vi "ArrayPadraoSuper.vi"(1 "VI":path, 3 "Array_TAGS/Config":string[](array[string])=["KPS-EVC-001", "KPS-EVC-002", "KPS-EVC-003", "KPS-EVC-004", "KPS-EVC-005", "KPS-EVC-006", "KPS-EVC-007", "KPS-EVC-008", "WPS-EVC-001", "WPS-EVC-002", "WPS-EVC-003", "WPS-EVC-004", "WPS-EVC-005", "WPS-EVC-006", "WPS-EVC-007", "WPS-EVC-008", "AMS-EVC-001B", "AMS-EVC-003A", "FIS-EVC-031", "FIS-EVC-011", "FIS-EVC-012", "FIS-EVC-021", "FIS-EVC-022", "FIS-EVC-001", "FIS-EVC-002", "KMS-EVC-001", "WMS-EVC-001A", "WMS-EVC-001B", "AMS-EVC-001C", "DG-EVC-001", "DG-EVC-ALL", "KPS-WR-ON", "WPS-WR-ON", "KPS-WR-OFF", "WPS-WR-OFF", "AMS-EVC-001A", "AMS-PY-005A", "AMS-FY-004A", "WMS-FCV-001", "KMS-FCV-001", "SPK-WR-VEL", "SPW-WR-VEL", "SKM-FIC-COR-KF-MAX", "SKM-FIC-COR-KF-MIN", "SKM-FIC-COR-WF-MAX", "SKM-FIC-COR-WF-MIN", "FSS-EVC-801", "FSS-EVC-802", "FSS-EVC-803", "CP-Y-601D", "CP-Y-601H", "FSS-EVC-804", "SHD-CV-HD", "SHD-CV-ALV", "SHD-ON-OFF", "FSS-EVC-805", "FSS-EVC-806", "DG-FCV-801", "Aplicação apenas de Leitura ??", "SALVAR/AQUISITAR", "KPS-FCV-001-W", "WPS-FCV-001-W"]) -> ()   [LabVIEW 2019]
uses:
  <vilib>/Utility/miscctls.llb/LVForegroundBackgroundColorsTypeDef.ctl
  <vilib>/Utility/miscctls.llb/LVTextColorsTypeDef.ctl
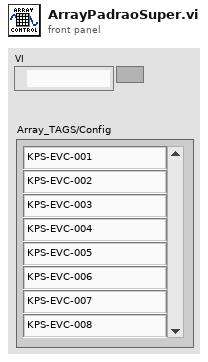
[diagram p1: front panel]
types:
  T1 = typedef "LVTextColorsTypeDef.ctl" = cluster{"Text Color":u32, "Background Color":u32}
  T2 = typedef "LVForegroundBackgroundColorsTypeDef.ctl" = cluster{"Foreground Color":u32, "Background Color":u32}
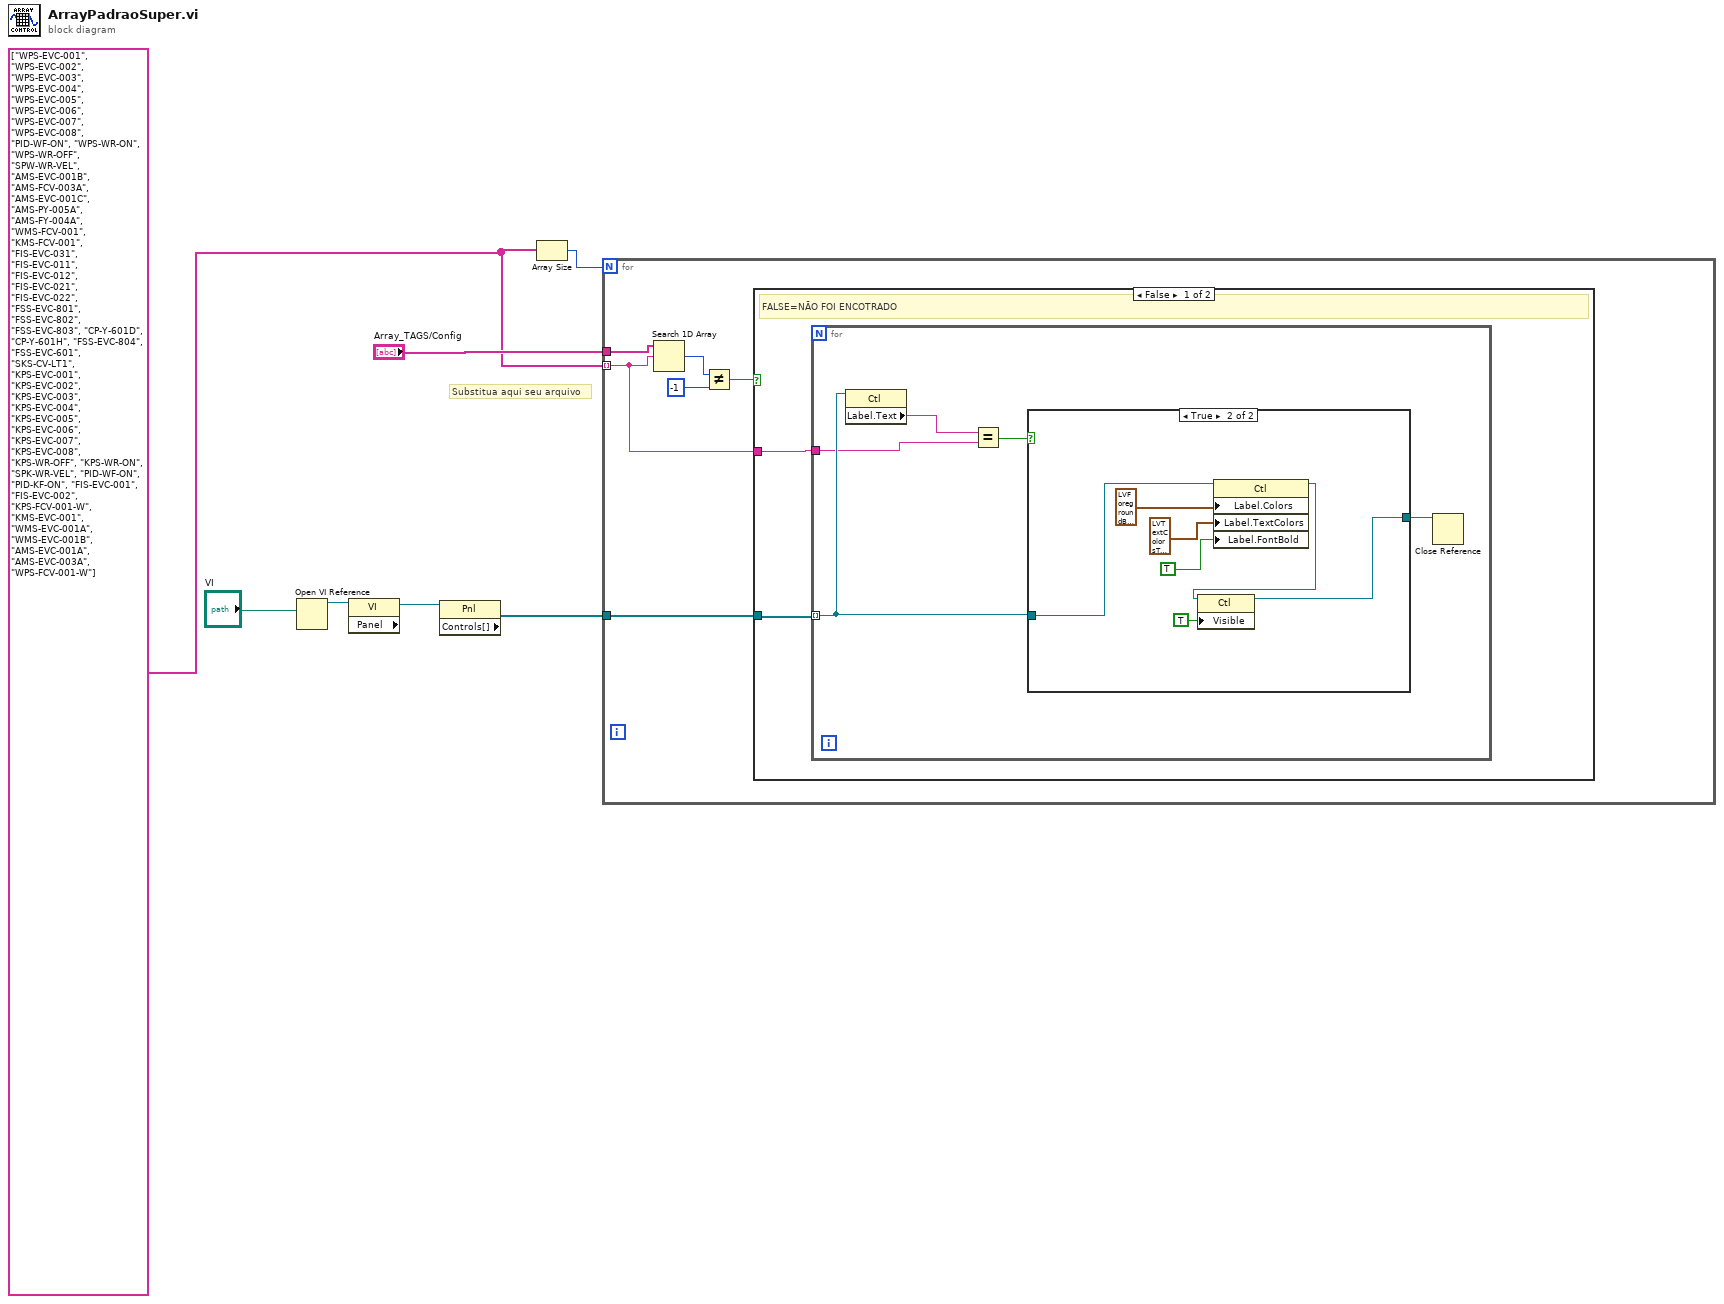
[diagram p0: block diagram]
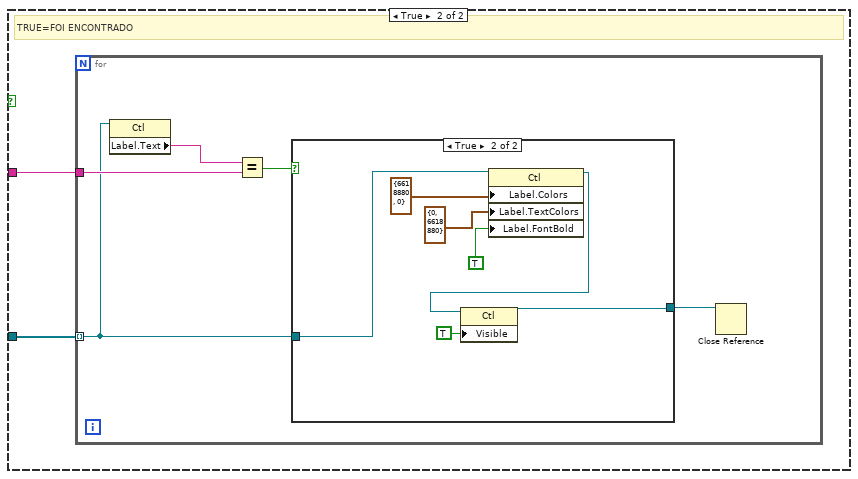
[diagram p3: hidden frame]
diagram:
  w1 = string[] ["WPS-EVC-001", "WPS-EVC-002", "WPS-EVC-003", "WPS-EVC-004", "WPS-EVC-005", "WPS-EVC-006", "WPS-EVC-007", "WPS-EVC-008", "PID-WF-ON", "WPS-WR-ON", "WPS-WR-OFF", "SPW-WR-VEL", "AMS-EVC-001B", "AMS-FCV-003A", "AMS-EVC-001C", "AMS-PY-005A", "AMS-FY-004A", "WMS-FCV-001", "KMS-FCV-001", "FIS-EVC-031", "FIS-EVC-011", "FIS-EVC-012", "FIS-EVC-021", "FIS-EVC-022", "FSS-EVC-801", "FSS-EVC-802", "FSS-EVC-803", "CP-Y-601D", "CP-Y-601H", "FSS-EVC-804", "FSS-EVC-601", "SKS-CV-LT1", "KPS-EVC-001", "KPS-EVC-002", "KPS-EVC-003", "KPS-EVC-004", "KPS-EVC-005", "KPS-EVC-006", "KPS-EVC-007", "KPS-EVC-008", "KPS-WR-OFF", "KPS-WR-ON", "SPK-WR-VEL", "PID-WF-ON", "PID-KF-ON", "FIS-EVC-001", "FIS-EVC-002", "KPS-FCV-001-W", "KMS-EVC-001", "WMS-EVC-001A", "WMS-EVC-001B", "AMS-EVC-001A", "AMS-EVC-003A", "WPS-FCV-001-W"] ("Array - String")
  # "Substitua aqui seu arquivo"
  n1 = Open VI Reference(vi path="VI") -> (vi reference=w6:refnum<vi>)  [unwired: 5 in, 1 out]
  n2 = property class="VI"(reference=w6) -> ("Panel"=w5:refnum<vi>)  [unwired: 1 in, 2 out]
  n3 = property class="Pnl"(reference=w5) -> ("Controls[]"=w4:refnum<vi>[])  [unwired: 1 in, 2 out]
  n4 = Array Size(array=w1) -> (size(s)=w7:i32)
  n5 = for {
    N: w7 -> [_]
    tunnel: w4 -> [w11]
    tunnel: "Array_TAGS/Config" -> [w10]
    tunnel: w1 -> [w8] mode=indexing
    n6 = Search 1D Array(1D array=w10, element=w8) -> (index of element=w13:i32)  [unwired: 1 in]
    n7 = Not Equal?(x=w13, y=-1) -> (x != y?=w9:bool)
    n8 = case shown="False" w9 {
      tunnel: w11 -> [w14 w30]
      tunnel: w8 -> [w15 w29]
      frame False {
        # "FALSE=NÃO FOI ENCOTRADO"
        n9 = for {
          tunnel: w14 -> [w20] mode=indexing
          tunnel: w15 -> [w17]
          n10 = property class="Ctl"(reference=w20) -> ("Label.Text"=w18:string)  [unwired: 1 in, 2 out]
          n11 = Equal?(x=w18, y=w17) -> (x = y?=w19:bool)
          n12 = case shown="True" w19 {
            tunnel: w20 -> [w21 w23]
            tunnel: [w21 w24] -> w16
            frame False {
            }
            frame True {
              n13 = property class="Ctl"(reference=w23, "Label.Colors"=T2 {"Foreground Color"=16711680, "Background Color"=16448250}, "Label.TextColors"=T1 {"Text Color"=16448250, "Background Color"=16711680} ("Label.Text Colors"), "Label.FontBold"=TRUE ("Label.Font:Bold")) -> (reference out=w22:refnum<vi>)  [unwired: 1 in, 1 out]
              n14 = property class="Ctl"(reference=w22, "Visible"=TRUE) -> (reference out=w24:refnum<vi>)  [unwired: 1 in, 1 out]
            }
          }
          n15 = Close Reference(reference=w16) -> ()  [unwired: 1 in, 1 out]
        }
      }
      frame True {
        # "TRUE=FOI ENCONTRADO"
        n16 = for {
          tunnel: w30 -> [w32] mode=indexing
          tunnel: w29 -> [w33]
          n17 = property class="Ctl"(reference=w32) -> ("Label.Text"=w34:string)  [unwired: 1 in, 2 out]
          n18 = Equal?(x=w34, y=w33) -> (x = y?=w35:bool)
          n19 = case shown="True" w35 {
            tunnel: w32 -> [w36 w39]
            tunnel: [w36 w38] -> w31
            frame False {
            }
            frame True {
              n20 = property class="Ctl"(reference=w39, "Label.Colors"=T2 {"Foreground Color"=6618880, "Background Color"=0}, "Label.TextColors"=T1 {"Text Color"=0, "Background Color"=6618880} ("Label.Text Colors"), "Label.FontBold"=TRUE ("Label.Font:Bold")) -> (reference out=w37:refnum<vi>)  [unwired: 1 in, 1 out]
              n21 = property class="Ctl"(reference=w37, "Visible"=TRUE) -> (reference out=w38:refnum<vi>)  [unwired: 1 in, 1 out]
            }
          }
          n22 = Close Reference(reference=w31) -> ()  [unwired: 1 in, 1 out]
        }
      }
    }
  }
